vi "ShowMessage.vi"(10 "字符串":string, 11 "Str引用句柄":refnum<vi>) -> ()   [LabVIEW 2012]
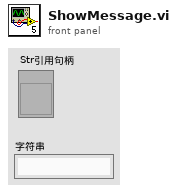
[diagram p1: front panel]
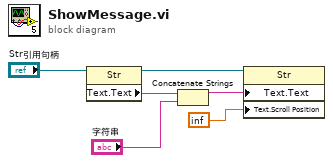
[diagram p0: block diagram]
diagram:
  n1 = property class="Str"(reference="Str引用句柄") -> (reference out=w5:refnum<vi>, "Text.Text"=w4:string)  [unwired: 1 in, 1 out]
  n2 = Concatenate Strings(w4, "字符串") -> (w2:string)
  n3 = property class="Str"(reference=w5, "Text.Text"=w2, "Text.Scroll Position"=inf) -> ()  [unwired: 1 in, 2 out]
